vi "Write Subtract BG.vi"(8 "error in (no error)":errorcluster, 10 "Subtract":bool, 11 "HIJ Vision App IMAQdx Display in":refnum<class "HIJ Vision App IMAQdx Display.lvclass">) -> (0 "error out":errorcluster, 3 "HIJ Vision App IMAQdx Display out":refnum<class "HIJ Vision App IMAQdx Display.lvclass">)   [LabVIEW 2020, in "HIJ Vision App IMAQdx Display.lvlib" / "HIJ Vision App IMAQdx Display.lvclass"]
uses:
  HIJ Vision App IMAQdx Display.lvclass
  HIJ Vision App IMAQdx Display.lvclass/HIJ Vision App IMAQdx Display.ctl
  Display Actors/HIJ IMAQdx Display/HIJ IMAQdx Display Messages/Write SubstractBG_ Msg/Write SubstractBG_ Msg.lvclass
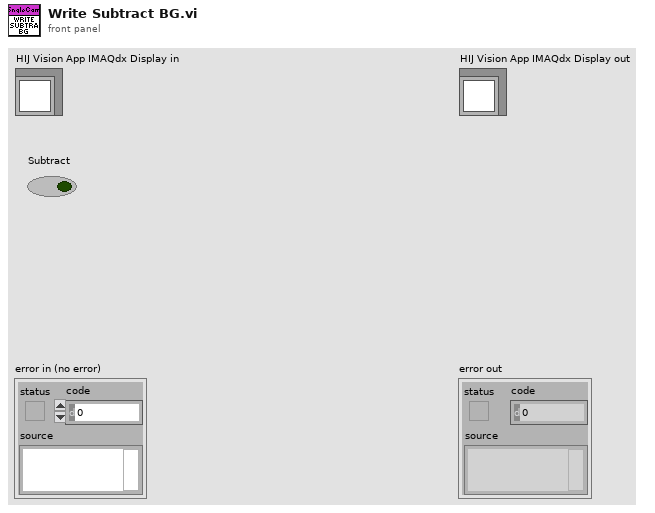
[diagram p1: front panel]
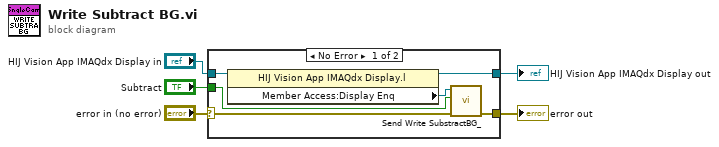
[diagram p0: block diagram]
diagram:
  n1 = case shown="No Error" "error in (no error)" {
    selector: "error in (no error)" -> [w7 w13]
    tunnel: [w6 w13] -> w4
    tunnel: [w10 w12] -> w2
    tunnel: "HIJ Vision App IMAQdx Display in" -> [w11 w12]
    tunnel: "Subtract" -> [w8 _]
    frame No Error {
      n2 = property class="HIJ Vision App IMAQdx Display.l"(reference=w11) -> (reference out=w10:refnum<class "HIJ Vision App IMAQdx Display.lvclass">, "Member Access:Display Enq"=w9:refnum<class "Message Enqueuer.lvclass">)  [unwired: 1 in, 1 out]
      n3 = call "Send Write SubstractBG_.vi"("error in (no error)"=w7, "SubstractBG?"=w8, "Message Enqueuer"=w9) -> ("error out"=w6:errorcluster)  [unwired: 7 in, 1 out]
    }
    frame Error {
    }
  }
  "error out" <- w4
  "HIJ Vision App IMAQdx Display out" <- w2
